vi "Match string in array.vi"(10 "String":string, 11 "String Array":string[](array[string])) -> (1 "Found":bool, 2 "Index":i32, 3 "Match":string)   [LabVIEW 2019]
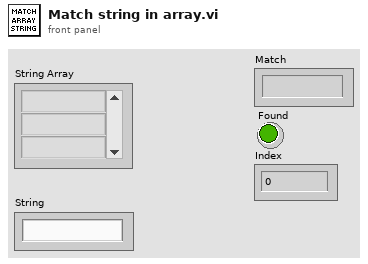
[diagram p1: front panel]
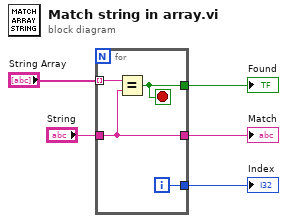
[diagram p0: block diagram]
diagram:
  n1 = for {
    tunnel: [w9] -> w2
    tunnel: [w8] -> w3
    tunnel: "String Array" -> [w7] mode=indexing
    tunnel: "String" -> [w6]
    tunnel: [w6] -> w1
    i -> [w9]
    stop <- w8 stop-if-true
    n2 = Equal?(x=w7, y=w6) -> (x = y?=w8:bool)
  }
  "Found" <- w3
  "Index" <- w2
  "Match" <- w1
